vi "sous-vi-registre-d‚calage2‚.vi"(0 "Cluster traitement":T3, 7 "entrée erreur":errorcluster caption="erreur entrée", 11 "Cluster":T2) -> (1 "Cluster en sortie":T1, 2 "taille (S1)":u32, 3 "taille (S2)":u32, 4 "S1":cluster{"X (S1;b1)":u32, "Y (S1;b1)":u32}, 6 "S2":cluster{"X (S1;b2) ":u32, "Y (S1;b2)":u32}, 8 "constante d'erreur":errorcluster caption="sortie erreur", 10 "S3":cluster{"X (S2;b1) ":u32, "Y (S2;b1)":u32}, 12 "Distance entre la caméra et le drone":dbl format="%#_4g", 13 "taille (S4)":u32, 14 "taille (S3)":u32, 15 "S4":cluster{"X (S2;b2)":u32, "Y (S2;b2)":u32})   [LabVIEW 2013]
panel:
  out "D4":dbl format="%#_13g"
  out "D3":dbl format="%#_13g"
  out "D2":dbl format="%#_13g"
  out "D1":dbl format="%#_13g"
  out "y4":u32
  out "x4":u32
  out "y3":u32
  out "x3":u32
  out "y2":u32
  out "x2":u32
  out "y1":u32
  out "x1":u32
  # "Ce sous-vi permet de laisser la dernière position connue de la signature en question si la \ntaille correspondante est nulle c'est à dire que plus rien n'est observé et de calculer \nla distance de l'objet à la caméra ci celui ci est présent."
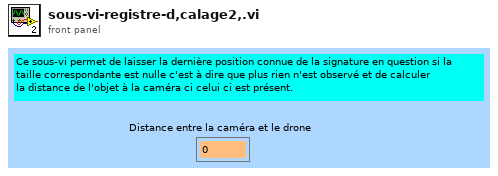
[diagram p1: front panel]
types:
  T1 = cluster{cluster{"taille (S1)":u32, "S1":cluster{"X (S2;b1) ":u32, "Y (S2;b1)":u32}}, cluster{"taille (S2)":u32, "S2":cluster{"X (S2;b1) ":u32, "Y (S2;b1)":u32}}, cluster{"taille (S3)":u32, "S3":cluster{"X (S2;b1) ":u32, "Y (S2;b1)":u32}}, cluster{"taille (S4)":u32, "S4":cluster{"X (S2;b1) ":u32, "Y (S2;b1)":u32}}}
  T2 = cluster{cluster{u32, cluster{u32, u32}}, cluster{u32, cluster{u32, u32}}, cluster{u32, cluster{u32, u32}}, cluster{u32, cluster{u32, u32}}}
  T3 = cluster{"S1":cluster{"X (S2;b1) ":u32, "Y (S2;b1)":u32}, "S2":cluster{"X (S2;b1) ":u32, "Y (S2;b1)":u32}, "S3":cluster{"X (S2;b1) ":u32, "Y (S2;b1)":u32}, "S4":cluster{"X (S2;b1) ":u32, "Y (S2;b1)":u32}, "taille (S1)":u32, "taille (S2)":u32, "taille (S3)":u32, "taille (S4)":u32}
  T4 = cluster{"taille (S1)":u32, "S1":cluster{"X (S2;b1) ":u32, "Y (S2;b1)":u32}}
  T5 = cluster{"taille (S2)":u32, "S2":cluster{"X (S2;b1) ":u32, "Y (S2;b1)":u32}}
  T6 = cluster{"taille (S4)":u32, "S4":cluster{"X (S2;b1) ":u32, "Y (S2;b1)":u32}}
  T7 = cluster{"taille (S3)":u32, "S3":cluster{"X (S2;b1) ":u32, "Y (S2;b1)":u32}}
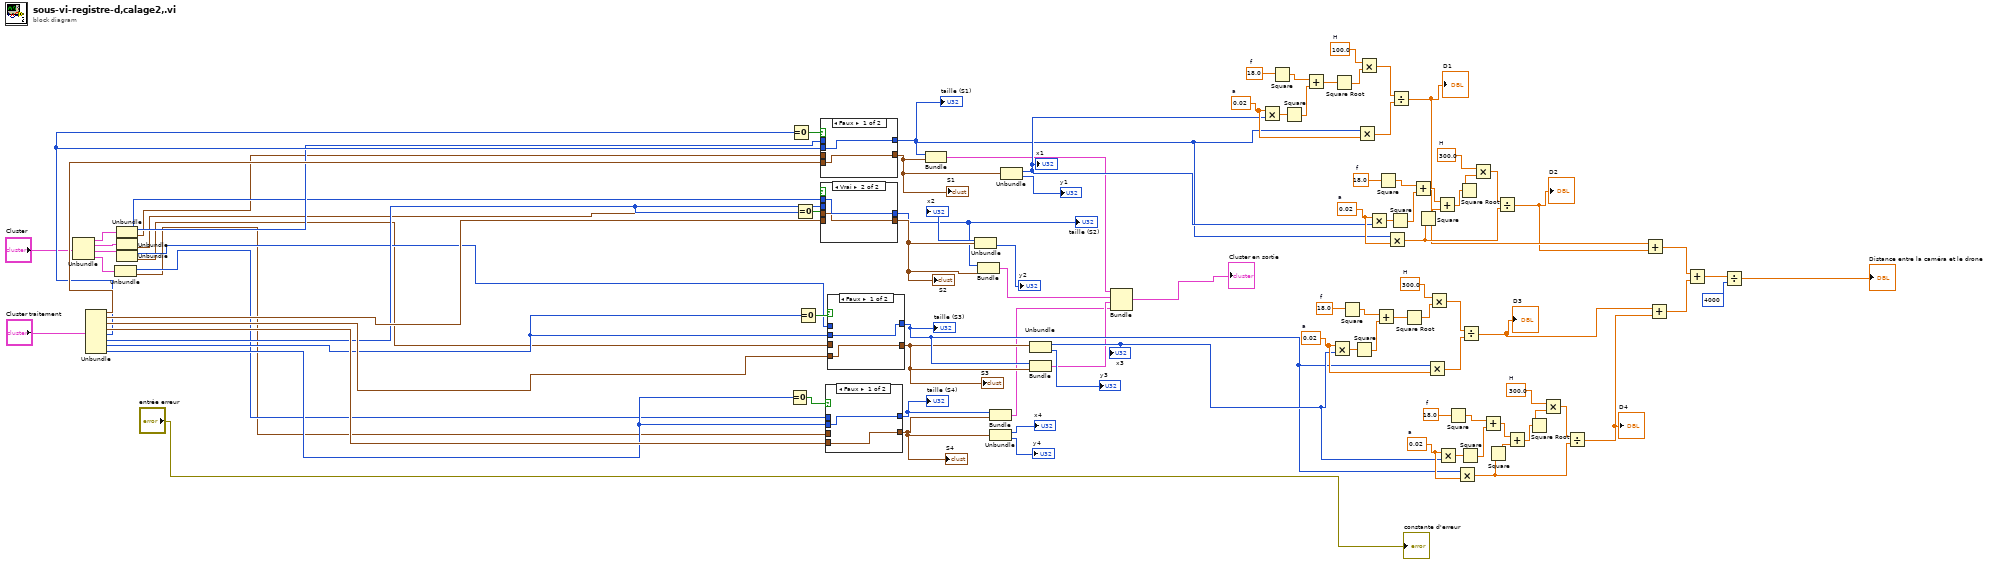
[diagram p0: block diagram]
diagram:
  w49 = 18.0  # f
  w42 = 0.02  # a
  w45 = 300.0  # H
  w59 = 18.0  # f
  w51 = 0.02  # a
  w54 = 300.0  # H
  w71 = 18.0  # f
  w64 = 0.02  # a
  w67 = 300.0  # H
  w81 = 18.0  # f
  w73 = 0.02  # a
  w76 = 100.0  # H
  n1 = Unbundle("Cluster") -> (w26:cluster{u32, cluster{u32, u32}}, w25:cluster{u32, cluster{u32, u32}}, w24:cluster{u32, cluster{u32, u32}}, w23:cluster{u32, cluster{u32, u32}})
  n2 = Unbundle("Cluster traitement") -> ("S1"=w95:cluster{"X (S2;b1) ":u32, "Y (S2;b1)":u32}, "S2"=w94:cluster{"X (S2;b1) ":u32, "Y (S2;b1)":u32}, "S3"=w93:cluster{"X (S2;b1) ":u32, "Y (S2;b1)":u32}, "S4"=w92:cluster{"X (S2;b1) ":u32, "Y (S2;b1)":u32}, "taille (S1)"=w90:u32, "taille (S2)"=w91:u32, "taille (S3)"=w89:u32, "taille (S4)"=w88:u32)
  n3 = Unbundle(w23) -> (w19:u32, w15:cluster{u32, u32})
  n4 = Unbundle(w26) -> (w22:u32, w18:cluster{u32, u32})
  n5 = Unbundle(w25) -> (w21:u32, w17:cluster{u32, u32})
  n6 = Unbundle(w24) -> (w20:u32, w16:cluster{u32, u32})
  n7 = Equal To 0?(x=w88) -> (x = 0?=w101:bool)
  n8 = Equal To 0?(x=w90) -> (x = 0?=w98:bool)
  n9 = Equal To 0?(x=w91) -> (x = 0?=w99:bool)
  n10 = Equal To 0?(x=w89) -> (x = 0?=w100:bool)
  n11 = case shown="Faux" w98 {
    tunnel: w22 -> [_ w105]
    tunnel: [w103 w105] -> w7
    tunnel: w90 -> [w103 _]
    tunnel: w95 -> [w102 _]
    tunnel: w18 -> [_ w104]
    tunnel: [w102 w104] -> w8
    frame False {
    }
    frame True {
    }
  }
  "S1" <- w8
  "taille (S1)" <- w7
  n12 = case shown="Vrai" w99 {
    tunnel: [w106 w109] -> w9
    tunnel: w21 -> [_ w109]
    tunnel: w91 -> [w106 _]
    tunnel: w17 -> [_ w108]
    tunnel: w94 -> [w107 _]
    tunnel: [w107 w108] -> w11
    frame False {
    }
    frame True {
    }
  }
  "S2" <- w11
  "taille (S2)" <- w9
  n13 = case shown="Faux" w101 {
    tunnel: [w111 w113] -> w13
    tunnel: w19 -> [_ w113]
    tunnel: w88 -> [w111 _]
    tunnel: w15 -> [_ w112]
    tunnel: w92 -> [w110 _]
    tunnel: [w110 w112] -> w14
    frame False {
    }
    frame True {
    }
  }
  "S4" <- w14
  "taille (S4)" <- w13
  n14 = case shown="Faux" w100 {
    tunnel: w20 -> [_ w117]
    tunnel: [w115 w117] -> w12
    tunnel: w89 -> [w115 _]
    tunnel: w16 -> [_ w116]
    tunnel: [w114 w116] -> w10
    tunnel: w93 -> [w114 _]
    frame False {
    }
    frame True {
    }
  }
  "S3" <- w10
  "taille (S3)" <- w12
  n15 = Bundle("taille (S1)"=w7, "S1"=w8) -> (w6:T4)  [unwired: 1 in]
  n16 = Unbundle(w11) -> ("X (S2;b1)"=→"x2":u32, "Y (S2;b1)"=→"y2":u32)
  n17 = Bundle("taille (S2)"=w9, "S2"=w11) -> (w5:T5)  [unwired: 1 in]
  n18 = Bundle("taille (S4)"=w13, "S4"=w14) -> (w3:T6)  [unwired: 1 in]
  n19 = Unbundle(w14) -> ("X (S2;b1)"=→"x4":u32, "Y (S2;b1)"=→"y4":u32)
  n20 = Unbundle(w8) -> ("X (S2;b1)"=w28:u32, "Y (S2;b1)"=→"y1":u32)
  "x1" <- w28
  n21 = Unbundle(w10) -> ("X (S2;b1)"=w27:u32, "Y (S2;b1)"=→"y3":u32)
  "x3" <- w27
  n22 = Bundle("taille (S3)"=w12, "S3"=w10) -> (w4:T7)  [unwired: 1 in]
  n23 = Bundle(w6, w5, w4, w3) -> (→"Cluster en sortie":T1)  [unwired: 1 in]
  n24 = Multiply(x=w73, y=w28) -> (x*y=w79:dbl)
  n25 = Square(x=w81) -> (x^2=w80:dbl)
  n26 = Square(x=w79) -> (x^2=w78:dbl)
  n27 = Add(x=w80, y=w78) -> (x+y=w77:dbl)
  n28 = Multiply(x=w51, y=w27) -> (x*y=w57:dbl)
  n29 = Square Root(x=w77) -> (sqrt(x)=w75:dbl)
  n30 = Square(x=w59) -> (x^2=w58:dbl)
  n31 = Square(x=w57) -> (x^2=w56:dbl)
  n32 = Multiply(x=w7, y=w73) -> (x*y=w72:dbl)
  n33 = Multiply(x=w76, y=w75) -> (x*y=w74:dbl)
  n34 = Multiply(x=w64, y=w28) -> (x*y=w69:dbl)
  n35 = Add(x=w58, y=w56) -> (x+y=w55:dbl)
  n36 = Square(x=w71) -> (x^2=w70:dbl)
  n37 = Multiply(x=w7, y=w64) -> (x*y=w62:dbl)
  n38 = Square(x=w69) -> (x^2=w68:dbl)
  n39 = Divide(x=w74, y=w72) -> (x/y=w37:dbl)
  "D1" <- w37
  n40 = Square Root(x=w55) -> (sqrt(x)=w53:dbl)
  n41 = Add(x=w70, y=w68) -> (x+y=w63:dbl)
  n42 = Square(x=w62) -> (x^2=w61:dbl)
  n43 = Multiply(x=w12, y=w51) -> (x*y=w50:dbl)
  n44 = Multiply(x=w54, y=w53) -> (x*y=w52:dbl)
  n45 = Add(x=w63, y=w61) -> (x+y=w60:dbl)
  n46 = Multiply(x=w42, y=w27) -> (x*y=w47:dbl)
  n47 = Square(x=w49) -> (x^2=w48:dbl)
  n48 = Multiply(x=w12, y=w42) -> (x*y=w40:dbl)
  n49 = Square Root(x=w60) -> (sqrt(x)=w66:dbl)
  n50 = Square(x=w47) -> (x^2=w46:dbl)
  n51 = Divide(x=w52, y=w50) -> (x/y=w35:dbl)
  "D3" <- w35
  n52 = Multiply(x=w67, y=w66) -> (x*y=w65:dbl)
  n53 = Add(x=w48, y=w46) -> (x+y=w41:dbl)
  n54 = Square(x=w40) -> (x^2=w39:dbl)
  n55 = Divide(x=w65, y=w62) -> (x/y=w36:dbl)
  "D2" <- w36
  n56 = Add(x=w41, y=w39) -> (x+y=w38:dbl)
  n57 = Square Root(x=w38) -> (sqrt(x)=w44:dbl)
  n58 = Multiply(x=w45, y=w44) -> (x*y=w43:dbl)
  n59 = Divide(x=w43, y=w40) -> (x/y=w34:dbl)
  "D4" <- w34
  n60 = Add(x=w37, y=w36) -> (x+y=w33:dbl)
  n61 = Add(x=w35, y=w34) -> (x+y=w32:dbl)
  n62 = Add(x=w33, y=w32) -> (x+y=w31:dbl)
  n63 = Divide(x=w31, y=4000) -> (x/y=→"Distance entre la caméra et le drone":dbl)
  "constante d'erreur" <- "entrée erreur"
